vi "append_image.vi"() -> ()   [LabVIEW 2014]
uses:
  <vilib>/printing/ReportDocExtensions.llb/Append Front Panel Image to Report (path).vi
  <vilib>/Utility/NIReport.llb/NI_ReportGenerationCore.lvlib
  <vilib>/Utility/NIReport.llb/NI_report.lvclass
panel:
  in  "template (empty)":path
  out "end out (Word)":i32
  out "start out (Word)":i32
  out "VI path out":path
  in  "visible area only?":bool
  in  "description":string
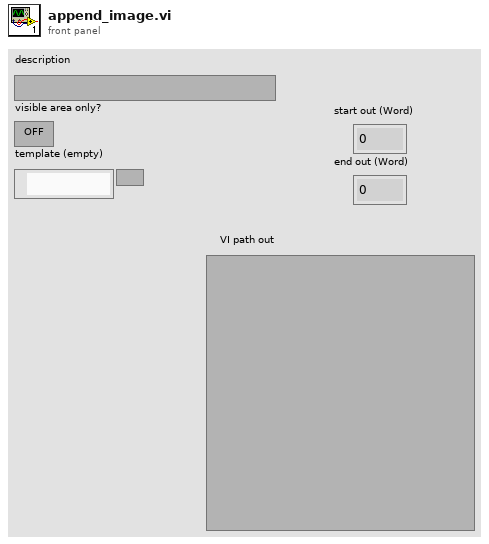
[diagram p1: front panel]
types:
  T1 = enum16{"Standard Report", "HTML", "Word", "Excel"}
  T2 = enum16{"maximized", "minimized", "normal", "no change"}
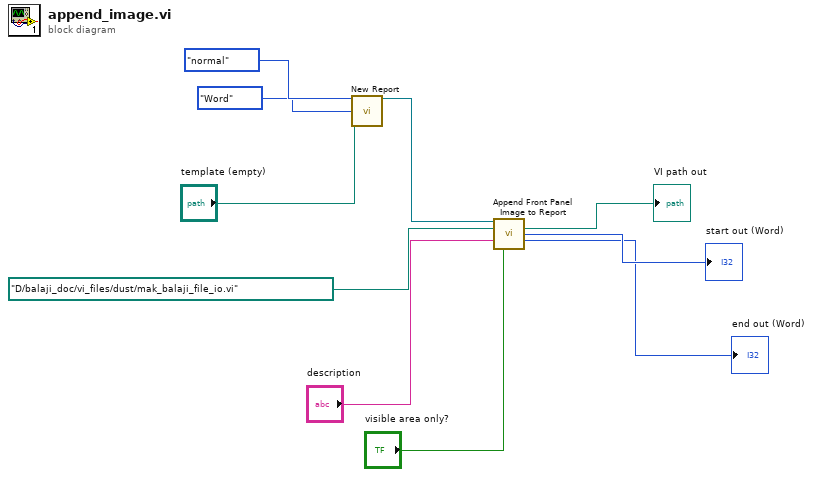
[diagram p0: block diagram]
diagram:
  n1 = call <vilib>:"New Report.vi"("window state (normal)"=T2."normal", "report type"=T1."Word", "template (empty)"="template (empty)") -> ("report out"=w2:refnum<class "NI_report.lvclass">)  [unwired: 11 in, 1 out]
  n2 = call-poly <vilib>:"Append Front Panel Image to Report.vi"("report in"=w2, "VI"=path "D:/balaji_doc/vi_files/dust/mak_balaji_file_io.vi", "description"="description", "visible area only?"="visible area only?") -> ("VI path out"=→"VI path out":path, "start out (Word)"=→"start out (Word)":i32, "end out (Word)"=→"end out (Word)":i32)  [unwired: 7 in, 2 out]
